vi "cube rotate up.vi"(8 "error in (no error)":errorcluster, 11 "cube in":T1) -> (0 "error out":errorcluster, 3 "cube out":T1)   [LabVIEW 2011]
uses:
  Typedef/cube.ctl
  Typedef/face.ctl
  Typedef/face rotate direction.ctl
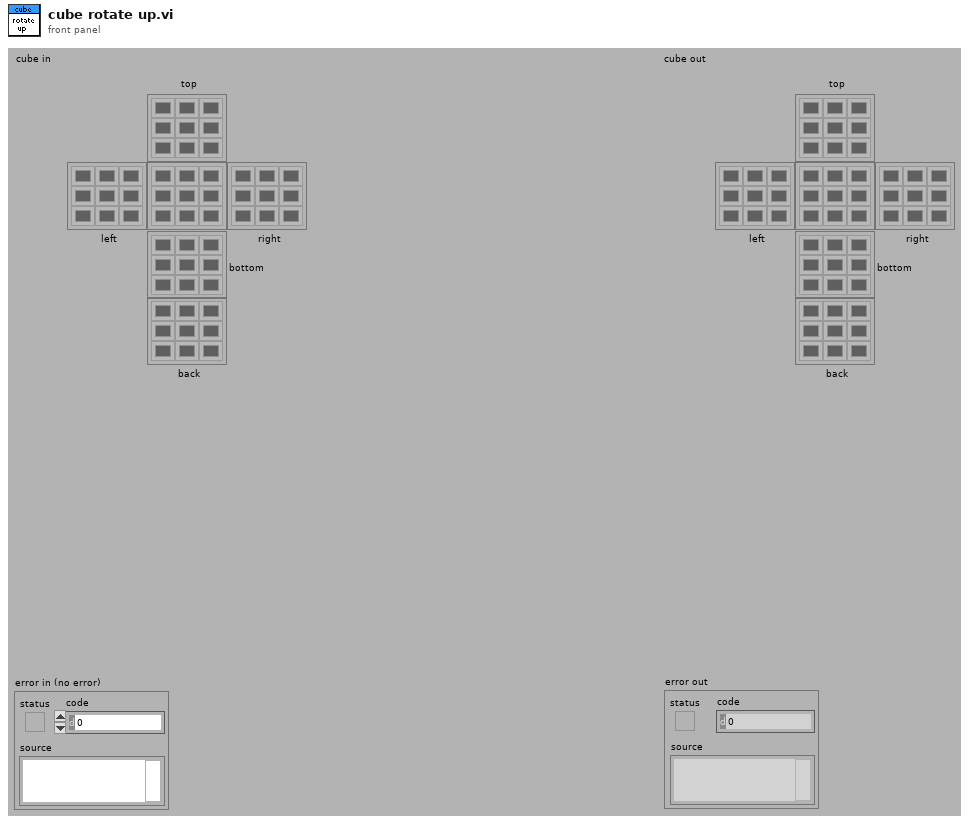
[diagram p1: front panel]
types:
  T1 = typedef "cube.ctl" = cluster{"top":T2, "left":T2, "right":T2, "bottom":T2, "back":T2, "front":T2}
  T2 = typedef "face.ctl" = u32[][]
  T3 = typedef "face rotate direction.ctl" = enum16{"+", "-"}
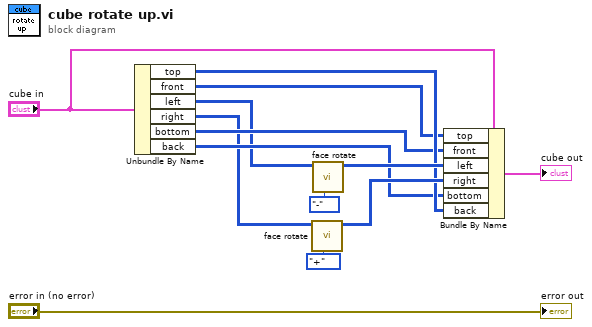
[diagram p0: block diagram]
diagram:
  n1 = Unbundle By Name("cube in") -> ("top"=w7:T2, "front"=w4:T2, "left"=w2:T2, "right"=w3:T2, "bottom"=w5:T2, "back"=w6:T2)
  n2 = call "face rotate.vi"("rotation directon"=face_rotate_direction."+", "face in"=w3) -> ("face out"=w9:T2)  [unwired: 8 in, 1 out]
  n3 = call "face rotate.vi"("rotation directon"=face_rotate_direction."-", "face in"=w2) -> ("face out"=w8:T2)  [unwired: 8 in, 1 out]
  n4 = Bundle By Name(cluster="cube in", "top"=w4, "front"=w5, "left"=w8, "right"=w9, "bottom"=w6, "back"=w7) -> (→"cube out":T1)
  "error out" <- "error in (no error)"
